vi "GetDigital.vi"(1 "Inst number":string, 2 "Array":cluster{"Inst #":string, "State":bool}[](array[cluster])) -> (0 "State":bool)   [LabVIEW 2020]
panel:
  # "When given a cluster array of instrument number/boolean pairs,\nreturns the state of the given instrument"
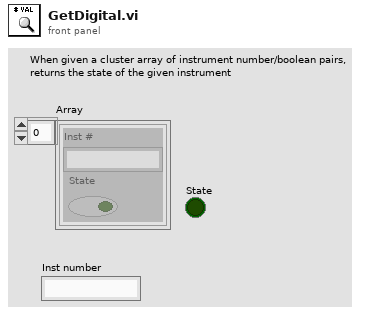
[diagram p1: front panel]
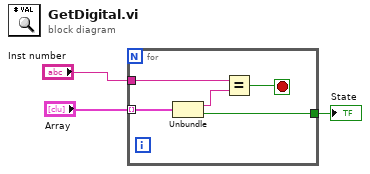
[diagram p0: block diagram]
diagram:
  n1 = for {
    tunnel: "Inst number" -> [w4]
    tunnel: "Array" -> [w8] mode=indexing
    tunnel: [w6] -> w1
    stop <- w7 stop-if-true
    n2 = Unbundle(w8) -> ("Inst #"=w5:string, "State"=w6:bool)
    n3 = Equal?(x=w4, y=w5) -> (x = y?=w7:bool)
  }
  "State" <- w1
